vi "Test_ConstructType_InvalidPath_Error.vi"(8 "error in (no error)":errorcluster, 11 "TestCase in":refnum<class "TestStreamToDiskTransport.lvclass">) -> (0 "error out":errorcluster, 3 "TestCase out":refnum<class "TestStreamToDiskTransport.lvclass">)   [LabVIEW 2017, in "TestStreamToDiskTransport.lvclass"]
uses:
  TestStreamToDiskTransport.lvclass
  Source/Concrete/StreamToDiskTransport/StreamToDiskTransport.lvclass/StreamToDiskTransport.ctl
  <vilib>/Utility/error.llb/Clear Errors.vi
  Source/Concrete/StreamToDiskTransport/StreamToDiskTransport.lvclass
panel:
  out "Return Error":errorcluster
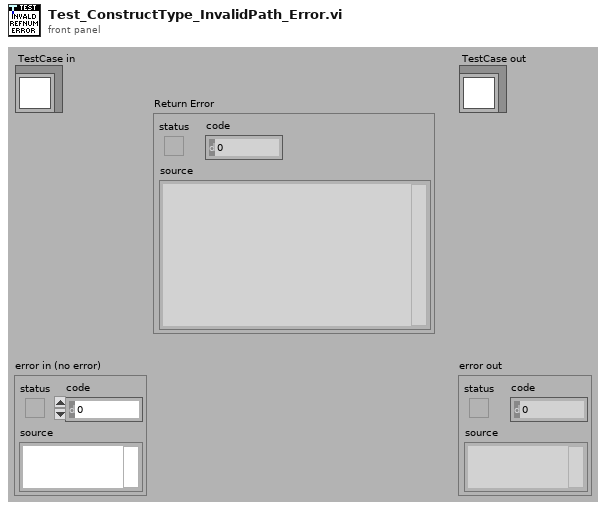
[diagram p1: front panel]
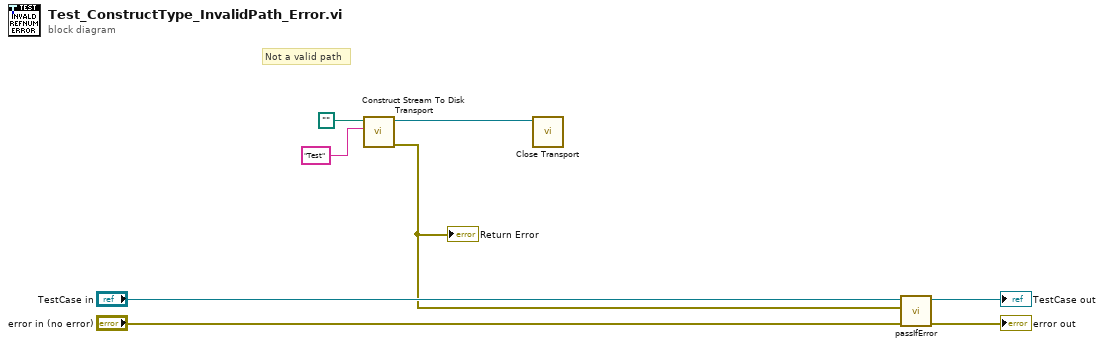
[diagram p0: block diagram]
diagram:
  # "Not a valid path"
  n1 = call "Construct Stream To Disk Transport.vi"("Channel Name"="Test" ("Key Name"), "File Path"=path "") -> ("error out"=w3:errorcluster, "StreamToDiskTransport"=w5:refnum<class "StreamToDiskTransport.lvclass">)  [unwired: 8 in]
  "Return Error" <- w3
  n2 = call-dynamic "Close Transport.vi"("StreamToDiskTransport"=w5) -> ()  [unwired: 10 in, 1 out]
  n3 = call-dynamic "passIfError.vi"("error in (no error)"="error in (no error)", "error"=w3, "TestCase in"="TestCase in") -> ("error out"=→"error out":errorcluster, "TestCase out"=→"TestCase out":refnum<class "TestStreamToDiskTransport.lvclass">)  [unwired: 7 in]
